vi "Identify and Replace Entire Element.vi"(7 "Named Cluster":variant, 8 "Identifying Attribute Value":string, 9 "Identifying Attribute Type":string, 10 "Element Type":string, 11 "XML String":string) -> (3 "Edited XML":string)   [LabVIEW 2019, in "EditSVG.lvclass"]
uses:
  EditSVG.lvclass
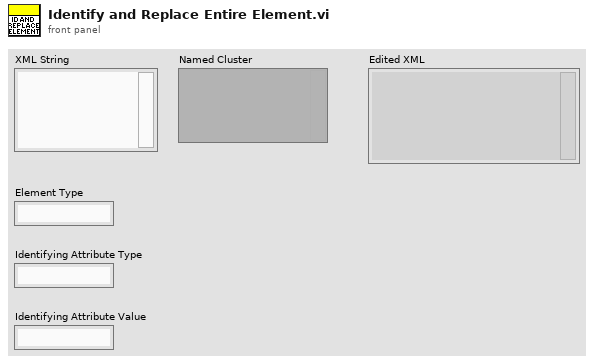
[diagram p1: front panel]
types:
  T1 = cluster{"width":string, "height":string, "preserveAspectRatio":string, "xlink:href":string, "id":string, "x":string, "y":string}
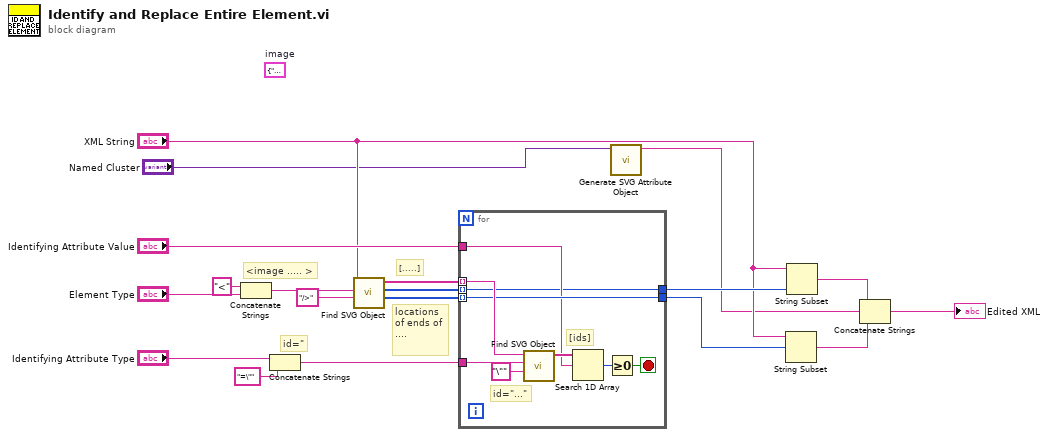
[diagram p0: block diagram]
diagram:
  (unwired) T1 {"width"="250", "height"="500", "preserveAspectRatio"="none", "xlink:href"="Mock%20Device2.jpg", "id"="image1-4", "x"="222", "y"="551"}  # image
  # "id=\""
  # "locations of ends of ...."
  # "[.....]"
  # "<image ..... >"
  n1 = Concatenate Strings("<" ("string"), "Element Type") -> (w13:string)
  n2 = Concatenate Strings("Identifying Attribute Type", "=\"" ("string")) -> (w16:string)
  n3 = call "Find SVG Object.vi"("Ending Delimiter"="/>", "Beginning Delimiter"=w13, "XML String"="XML String") -> ("Ending Indices"=w15:i32[], "Beginning Indices"=w9:i32[], "Found Values"=w18:string[])  [unwired: 6 in]
  n4 = for {
    tunnel: w18 -> [w28] mode=indexing
    tunnel: w16 -> [w26]
    tunnel: "Identifying Attribute Value" -> [w21]
    tunnel: w15 -> [w25] mode=indexing
    tunnel: [w25] -> w7
    tunnel: [w20] -> w8
    tunnel: w9 -> [w20] mode=indexing
    stop <- w22 stop-if-true
    # "id=\"...\""
    # "[ids]"
    n5 = call "Find SVG Object.vi"("Ending Delimiter"="\"", "Beginning Delimiter"=w26, "XML String"=w28) -> ("Found Values"=w24:string[])  [unwired: 6 in, 2 out]
    n6 = Search 1D Array(1D array=w24, element=w21) -> (index of element=w23:i32)  [unwired: 1 in]
    n7 = Greater Or Equal To 0?(x=w23) -> (x >= 0?=w22:bool)
  }
  n8 = call "Generate SVG Attribute Object.vi"("Named Cluster of Data"="Named Cluster") -> ("SVG Attribute Object"=w3:string)  [unwired: 9 in, 1 out]
  n9 = String Subset(string="XML String", offset (0)=w7) -> (substring=w4:string)  [unwired: 1 in]
  n10 = String Subset(string="XML String", length (rest)=w8) -> (substring=w5:string)  [unwired: 1 in]
  n11 = Concatenate Strings(w5, w3, w4) -> (→"Edited XML":string)
